vi "Write 1Ch NSamp (DBL).vi"(5 "timestamps":timestamp[](array[numeric]), 7 "index_channel":u32, 8 "error in":errorcluster, 9 "data":dbl[](array[numeric]), 10 "channel":u32, 11 "writer":u64) -> (0 "error out":errorcluster, 3 "writer out":u64)   [LabVIEW 2026, in "synnax_clib.lvlib"]
uses:
  synnax_clib.lvlib
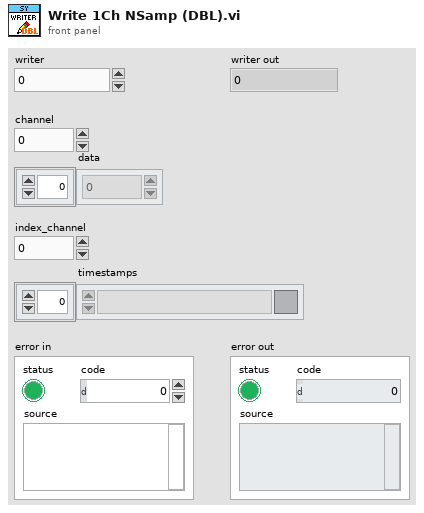
[diagram p1: front panel]
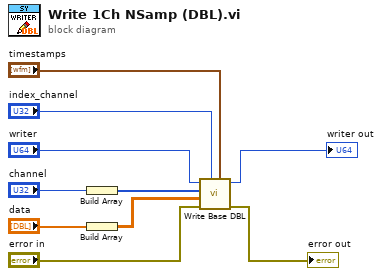
[diagram p0: block diagram]
diagram:
  n1 = Build Array("channel") -> (w5:u32[])
  n2 = Build Array("data") -> (w1:dbl[][])
  n3 = call "Write Base DBL.vi"("timestamps"="timestamps", "index_channel"="index_channel", "error in"="error in", "data"=w1, "channels"=w5, "writer"="writer") -> ("error out"=→"error out":errorcluster, "writer out"=→"writer out":u64)  [unwired: 4 in]
